vi "5afunctiongen.vi"() -> ()   [LabVIEW 2013]
uses:
  <vilib>/measure/NI_MABase.lvlib
panel:
  in  "signal type":T1(ring)
  out "Waveform Graph":waveform(dbl)(graph)
  in  "phse":dbl(knob) scale=0.0..360.0
  in  "frreq":dbl(knob) scale=0.0..100.0
  in  "amp":dbl(knob) scale=0.0..10.0 scale format="%#_10g"
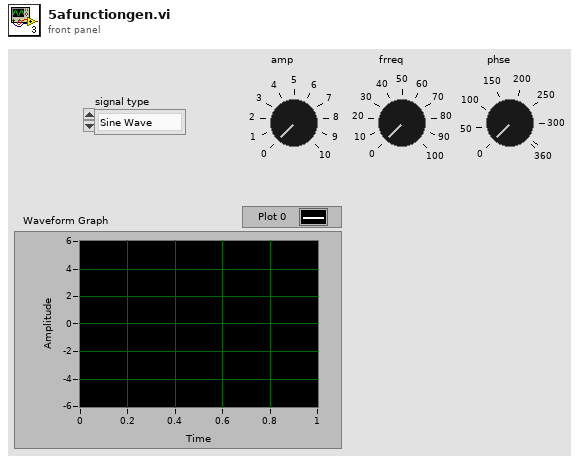
[diagram p1: front panel]
types:
  T1 = enum16{"Sine Wave", "Triangle Wave", "Square Wave", "Sawtooth Wave"}
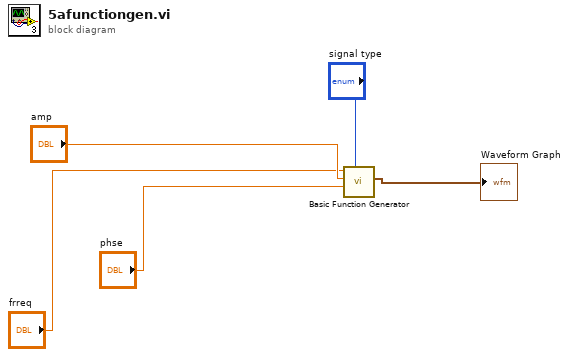
[diagram p0: block diagram]
diagram:
  n1 = call <vilib>:"Basic Function Generator.vi"("signal type"="signal type", "phase"="phse", "amplitude"="amp", "frequency"="frreq") -> ("signal out"=→"Waveform Graph":waveform(dbl))  [unwired: 5 in, 2 out]
